vi "启动整机测试 (子VI).vi"() -> (0 "error out":T1={"status"=FALSE, "代码"=4, "source"=""} caption="错误输出" {"代码" items=["执行成功"=1, "执行失败，但不知道原因"=2, "命令请求条件错误"=3, "通讯超时"=4, "系统繁忙不能执行"=5, "系统故障"=6, "没有数据"=100]})   [LabVIEW 2016]
uses:
  PLC/PLC.lvlib
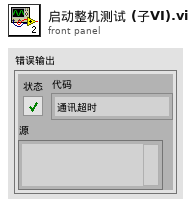
[diagram p1: front panel]
types:
  T1 = cluster{"status":bool, "代码":u16, "source":string}
  T2 = enum32{"Bad", "Idle", "Run top level", "Running"}
  T3 = cluster{"测试模式":enum16{"正常测试", "集成干预"}, "参数启用":cluster{"氨氮":bool, "总磷总氮":bool, "CODMn":bool, "CODcr":bool, "多参数":bool, "超标留样":bool}}
  T4 = cluster{"氨氮":bool, "总磷总氮":bool, "CODmn":bool, "CODCr":bool, "多参数":bool, "超标留样":bool}
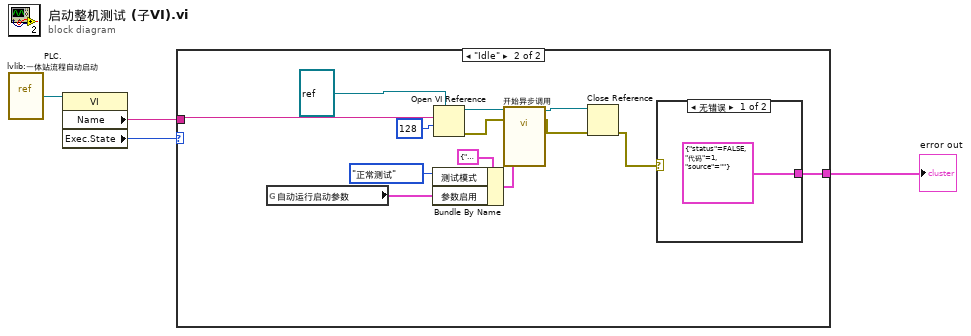
[diagram p0: block diagram]
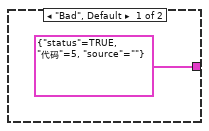
[diagram p2: hidden frame]
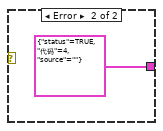
[diagram p3: hidden frame]
diagram:
  n1 = vi-ref "PLC.lvlib:一体站流程自动启动.vi"() -> (w3:refnum<vi>)
  n2 = property class="VI"(reference=w3) -> ("Name"=w4:string, "Exec.State"=w2:T2)  [unwired: 1 in, 2 out]
  n3 = case shown="\"Idle\"" w2 {
    tunnel: w4 -> [_ w13]
    tunnel: [T1 {"status"=TRUE, "代码"=5, "source"=""} ("error out") w11] -> w1
    frame "Bad", Default {
    }
    frame "Idle" {
      n4 = global read "系统设置全局变量.vi" "自动运行启动参数"() -> (w6:T4)
      n5 = Bundle By Name(cluster=T3 {"测试模式"=enum."正常测试", "参数启用"={"氨氮"=FALSE, "总磷总氮"=FALSE, "CODMn"=FALSE, "CODcr"=FALSE, "多参数"=FALSE, "超标留样"=FALSE}} ("参数"), "测试模式"=enum16{"正常测试", "集成干预", "加标回收"}."正常测试", "参数启用"=w6) -> (w7:T3)
      n6 = Open VI Reference(type specifier VI Refnum (for type only)=refnum<vi> refnum, vi path=w13, options=128 ("选项")) -> (vi reference=w15:refnum<vi>, error out=w17:errorcluster)  [unwired: 3 in]
      n7 = call-by-ref "开始异步调用"(reference=w15, error in=w17, "参数"=w7) -> (reference out=w16:refnum<vi>, error out=w18:errorcluster)  [unwired: 11 in]
      n8 = Close Reference(reference=w16, error in (no error)=w18) -> (error out=w10:errorcluster)
      n9 = case shown="无错误" w10 {
        tunnel: [T1 {"status"=FALSE, "代码"=1, "source"=""} ("error out") T1 {"status"=TRUE, "代码"=4, "source"=""} ("error out")] -> w11
        frame No Error {
        }
        frame Error {
        }
      }
    }
  }
  "error out" <- w1
